vi "Update.vi"(8 "error in (no error)":errorcluster, 11 "Snake in":refnum<class "Snake.lvclass">) -> (0 "error out":errorcluster, 3 "Snake out":refnum<class "Snake.lvclass">)   [LabVIEW 2019, in "RT_Game.lvlib" / "Snake.lvclass"]
uses:
  Snake.lvclass
  Snake.lvclass/Snake.ctl
  Game/Game.lvclass
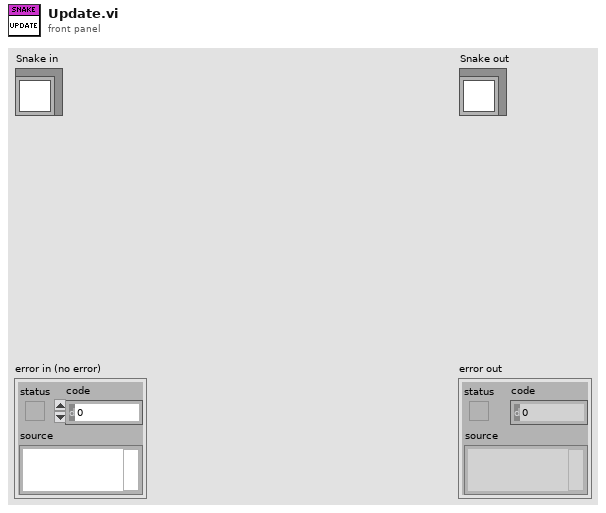
[diagram p1: front panel]
types:
  T1 = typedef "RT_Game.lvlib/Game.lvclass/Coordinate.ctl" = cluster{"x":i16, "y":i16}
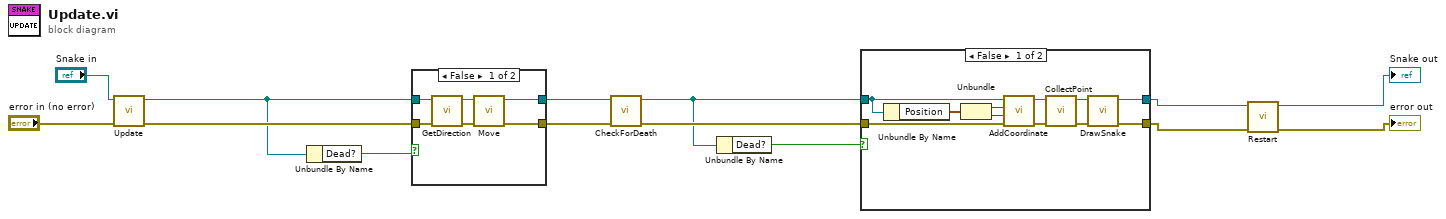
[diagram p0: block diagram]
diagram:
  n1 = call-parent "Update.vi"("error in (no error)"="error in (no error)", "Game in"="Snake in") -> ("error out"=w14:errorcluster, "Game out"=w4:refnum<class "Snake.lvclass">)  [unwired: 8 in]
  n2 = Unbundle By Name(w4) -> ("Dead?"=w3:bool)
  n3 = case shown="False" w3 {
    tunnel: w14 -> [w20 w21]
    tunnel: [w18 w21] -> w10
    tunnel: [w16 w22] -> w7
    tunnel: w4 -> [w15 w22]
    frame False {
      n4 = call "GetDirection.vi"("error in (no error)"=w20, "Snake in"=w15) -> ("error out"=w19:errorcluster, "Snake out"=w17:refnum<class "Snake.lvclass">)  [unwired: 8 in]
      n5 = call "Move.vi"("error in (no error)"=w19, "Snake in"=w17) -> ("error out"=w18:errorcluster, "Snake out"=w16:refnum<class "Snake.lvclass">)  [unwired: 8 in]
    }
    frame True {
    }
  }
  n6 = call "CheckForDeath.vi"("error in (no error)"=w10, "Snake in"=w7) -> ("error out"=w8:errorcluster, "Snake out"=w6:refnum<class "Snake.lvclass">)  [unwired: 8 in]
  n7 = Unbundle By Name(w6) -> ("Dead?"=w5:bool)
  n8 = case shown="False" w5 {
    tunnel: [w33 w34] -> w12
    tunnel: [w32 w35] -> w11
    tunnel: w8 -> [w29 w34]
    tunnel: w6 -> [w26 w35]
    frame False {
      n9 = Unbundle By Name(w26) -> ("Position"=w25:T1)
      n10 = Unbundle(w25) -> ("x"=w24:i16, "y"=w23:i16)
      n11 = call "AddCoordinate.vi"("error in (no error)"=w29, "y"=w23, "x"=w24, "Snake in"=w26) -> ("error out"=w28:errorcluster, "Snake out"=w27:refnum<class "Snake.lvclass">)  [unwired: 6 in]
      n12 = call "CollectPoint.vi"("error in (no error)"=w28, "Snake in"=w27) -> ("error out"=w30:errorcluster, "Snake out"=w31:refnum<class "Snake.lvclass">)  [unwired: 8 in]
      n13 = call "DrawSnake.vi"("error in (no error)"=w30, "Snake in"=w31) -> ("error out"=w33:errorcluster, "Snake out"=w32:refnum<class "Snake.lvclass">)  [unwired: 8 in]
    }
    frame True {
    }
  }
  n14 = call "Restart.vi"("error in (no error)"=w12, "Snake in"=w11) -> ("error out"=→"error out":errorcluster, "Snake out"=→"Snake out":refnum<class "Snake.lvclass">)  [unwired: 8 in]
